vi "waitTerminator.vi"(0 "HIFU UART in":refnum<visa-resource-name>, 1 "waitTime":dbl=10.0, 2 "error in (no error)":errorcluster) -> (3 "HIFU UART out":refnum<visa-resource-name>, 4 "OK?":bool, 5 "log":string, 6 "error out":errorcluster)   [LabVIEW 2016]
uses:
  <vilib>/regexp/Match Regular Expression.xnode
panel:
  out "Array":u32[](array[numeric])
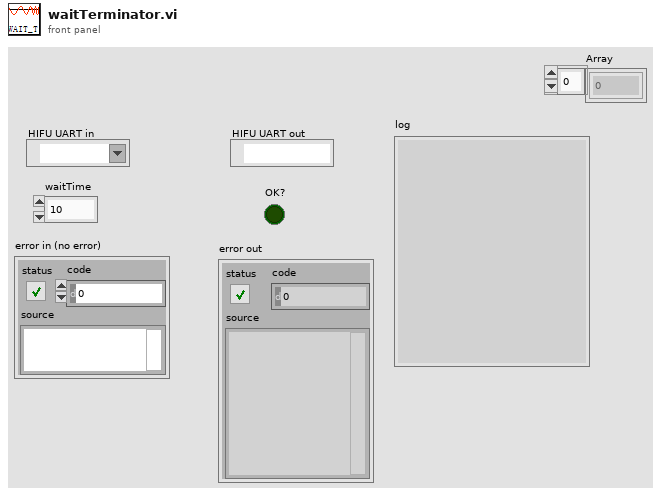
[diagram p1: front panel]
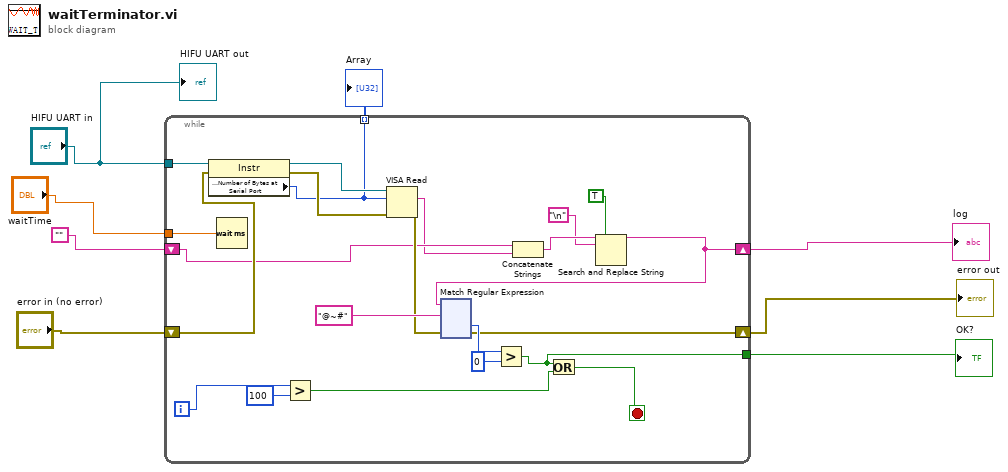
[diagram p0: block diagram]
diagram:
  n1 = while {
    tunnel: "HIFU UART in" -> [w30]
    shift-right: [w11] -> w4
    shift-left: "" -> [w16]
    shift-right: [w18] -> w2
    shift-left: "error in (no error)" -> [w29]
    tunnel: [w17] -> w6
    tunnel: "waitTime" -> [w14]
    tunnel: [w9] -> w1 mode=indexing
    i -> [w23]
    stop <- w20 stop-if-true
    n2 = property class="Instr"(reference=w30, error in=w29) -> (reference out=w28:refnum<visa-resource-name>, error out=w27:errorcluster, "Serial Settings:Number of Bytes at Serial Port"=w9:u32)
    n3 = Wait (ms)(milliseconds to wait=w14) -> ()  [unwired: 1 out]
    n4 = Greater?(x=w23, y=100) -> (0:w21:bool)
    n5 = VISA Read(VISA resource name=w28, byte count=w9, error in (no error)=w27) -> (read buffer=w15:string, error out=w19:errorcluster)  [unwired: 2 out]
    n6 = Concatenate Strings(w16, w15) -> (w13:string)
    n7 = Search and Replace String(replace all?=TRUE ("replace all? (F)"), input string=w13, search string="\n") -> (result string=w11:string)  [unwired: 5 in, 3 out]
    n8 = xnode "Match Regular Expression"("input string"=w11, "regular expression"="@~#", "error in"=w19) -> ("offset past match"=w25:i32, "error out"=w18:errorcluster)  [unwired: 3 in, 3 out]
    n9 = Greater?(x=w25, y=0) -> (0:w17:bool)
    n10 = Or(x=w17, y=w21) -> (x .or. y?=w20:bool)
  }
  "OK?" <- w6
  "log" <- w4
  "error out" <- w2
  "Array" <- w1
  "HIFU UART out" <- "HIFU UART in"
